vi "GatlingLoop.vi"(8 "error in":errorcluster) -> ()   [LabVIEW 2014]
uses:
  <vilib>/Rock Robotics/WPI/Relay/WPI_RelayValue.ctl
  <vilib>/Rock Robotics/WPI/Solenoid/WPI_SolenoidValue.ctl
  Robot Global Data.vi
  <vilib>/Rock Robotics/WPI/Solenoid/WPI_SolenoidSetEnum.vi
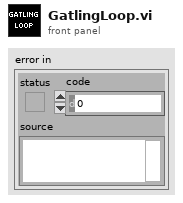
[diagram p1: front panel]
types:
  T1 = typedef "WPI_SolenoidValue.ctl" = enum16{"Off", "On", "Forward", "Reverse"}
  T2 = typedef "WPI_RelayValue.ctl" = enum16{"Off", "On", "Forward", "Reverse"}
  T3 = typedef "WPI_SolenoidDevRef.ctl" = cluster{"DevStatus":errorcluster, "Pneumatics Control Module":u8, "Forward Solenoid Channel":T4, "Reverse Solenoid Channel":T4}
  T4 = typedef "WPI_SolenoidChannel.ctl" = enum8{"Solenoid 0", "Solenoid 1", "Solenoid 2", "Solenoid 3", "Solenoid 4", "Solenoid 5", "Solenoid 6", "Solenoid 7", "Invalid"}
  T5 = typedef "WPI_MotorControlDeviceRef.ctl" = cluster{"DeviceStatus":errorcluster, "Type":T6, "PWM":cluster{"Controller":T7, "PWM Channel":T8, "DeadBand":T9}, "CAN":cluster{"Device Number":u8, "Control Mode":T10, "Semaphore":T11, "Max Vout":dbl, "TalonSRX Control Mode":T12}, "Invert":bool, "TransformRef":T13, "InvTransformRef":T13}
  T6 = typedef "WPI_MotorControlType.ctl" = enum16{"PWM", "CAN", "CANTalonSRX"}
  T7 = typedef "FPGA_TypedefDigitalModule.ctl" = enum16{"Controller 1"}
  T8 = typedef "FPGA_DIOPWMChannel.ctl" = enum8{"PWM 0", "PWM 1", "PWM 2", "PWM 3", "PWM 4", "PWM 5", "PWM 6", "PWM 7", "PWM 8", "PWM 9", "PWM MXP 0", "PWM MXP 1", "PWM MXP 2", "PWM MXP 3", "PWM MXP 4", "PWM MXP 5", "PWM MXP 6", "PWM MXP 7", "PWM MXP 8", "PWM MXP 9", "Invalid"}
  T9 = typedef "WPI_PWMDeadband.ctl" = cluster{"Name":string, "maxPositivePwm":i32, "minPositivePwm":i32, "centerPwm":i32, "maxNegativePwm":i32, "minNegativePwm":i32, "angularRange":u16}
  T10 = typedef "WPI_CANJaguar_ControlMode.ctl" = enum8{"Percent VBus", "Current", "Speed", "Position", "Voltage"}
  T11 = typedef "Semaphore RefNum" = refnum<k1>
  T12 = typedef "WPI_CANTalonSRX_APIControlMode.ctl" = enum8{"Percent VBus", "Speed", "Position", "Slave", "Unchanged / Invalid"}
  T13 = typedef "WPI_PWMTransform_ConPane.ctl" = refnum<vi>
  T14 = typedef "WPI_RelayDevRef.ctl" = cluster{"DevStatus":errorcluster, "Relay Channel":T15, "Controller":T7, "Relay Direction":T16}
  T15 = typedef "FPGA_DIORelayChannel.ctl" = enum8{"Relay 0", "Relay 1", "Relay 2", "Relay 3", "Invalid"}
  T16 = typedef "WPI_RelayDirection.ctl" = enum16{"Both directions", "Forward only", "Reverse only"}
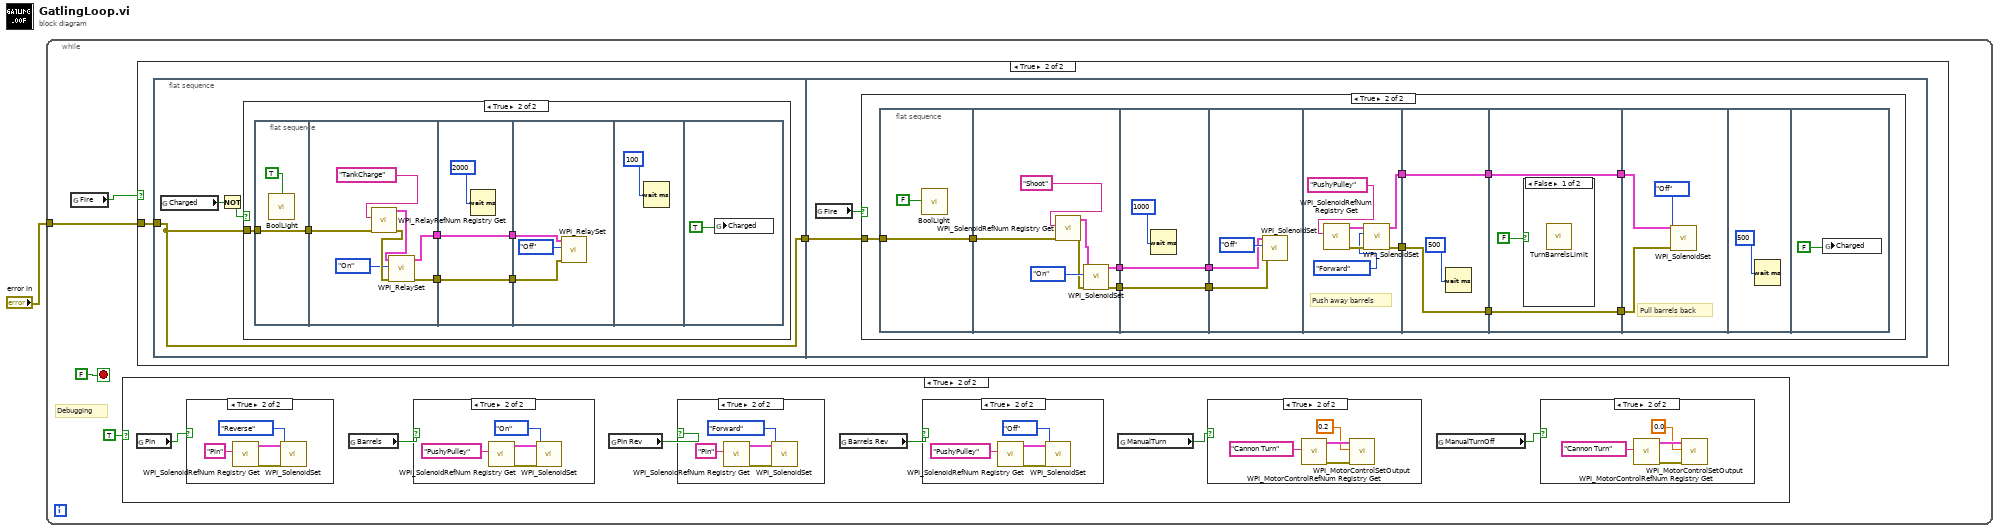
[diagram p0: block diagram]
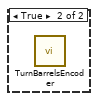
[diagram p12: hidden frame]
diagram:
  n1 = while {
    tunnel: "error in" -> [w3]
    stop <- FALSE stop-if-true
    # "Debugging"
    n2 = global read "Robot Global Data.vi" "Fire"() -> (w4:bool)
    n3 = case shown="True" TRUE {
      frame False {
      }
      frame True {
        n4 = global read "Robot Global Data.vi" "Pin"() -> (w11:bool)
        n5 = case shown="True" w11 {
          frame False {
          }
          frame True {
            n6 = call <vilib>:"WPI_SolenoidRefNum Registry Get.vi"("refnum name"="Pin") -> ("error out"=w34:errorcluster, "SolenoidDevRef"=w33:T3)  [unwired: 9 in]
            n7 = call-poly <vilib>:"WPI_SolenoidSet.vi"("error in (no error)"=w34, "Value"=WPI_SolenoidValue."Reverse", "SolenoidDevRef"=w33) -> ()  [unwired: 7 in, 2 out]
          }
        }
        n8 = global read "Robot Global Data.vi" "Barrels"() -> (w10:bool)
        n9 = case shown="True" w10 {
          frame False {
          }
          frame True {
            n10 = call <vilib>:"WPI_SolenoidRefNum Registry Get.vi"("refnum name"="PushyPulley") -> ("error out"=w30:errorcluster, "SolenoidDevRef"=w29:T3)  [unwired: 9 in]
            n11 = call-poly <vilib>:"WPI_SolenoidSet.vi"("error in (no error)"=w30, "Value"=WPI_SolenoidValue."On", "SolenoidDevRef"=w29) -> ()  [unwired: 7 in, 2 out]
          }
        }
        n12 = global read "Robot Global Data.vi" "Pin Rev"() -> (w9:bool)
        n13 = case shown="True" w9 {
          frame False {
          }
          frame True {
            n14 = call <vilib>:"WPI_SolenoidRefNum Registry Get.vi"("refnum name"="Pin") -> ("error out"=w26:errorcluster, "SolenoidDevRef"=w25:T3)  [unwired: 9 in]
            n15 = call-poly <vilib>:"WPI_SolenoidSet.vi"("error in (no error)"=w26, "Value"=WPI_SolenoidValue."Forward", "SolenoidDevRef"=w25) -> ()  [unwired: 7 in, 2 out]
          }
        }
        n16 = global read "Robot Global Data.vi" "Barrels Rev"() -> (w8:bool)
        n17 = case shown="True" w8 {
          frame False {
          }
          frame True {
            n18 = call <vilib>:"WPI_SolenoidRefNum Registry Get.vi"("refnum name"="PushyPulley") -> ("error out"=w22:errorcluster, "SolenoidDevRef"=w21:T3)  [unwired: 9 in]
            n19 = call-poly <vilib>:"WPI_SolenoidSet.vi"("error in (no error)"=w22, "Value"=WPI_SolenoidValue."Off", "SolenoidDevRef"=w21) -> ()  [unwired: 7 in, 2 out]
          }
        }
        n20 = global read "Robot Global Data.vi" "ManualTurn"() -> (w7:bool)
        n21 = case shown="True" w7 {
          frame False {
          }
          frame True {
            n22 = call <vilib>:"WPI_MotorControlRefNum Registry Get.vi"("refnum name"="Cannon Turn") -> ("error out"=w18:errorcluster, "MotorControlDevRef"=w17:T5)  [unwired: 9 in]
            n23 = call <vilib>:"WPI_MotorControlSetOutput.vi"("error in (no error)"=w18, "Output"=0.2, "MotorControlDevRef"=w17) -> ()  [unwired: 6 in, 3 out]
          }
        }
        n24 = global read "Robot Global Data.vi" "ManualTurnOff"() -> (w6:bool)
        n25 = case shown="True" w6 {
          frame False {
          }
          frame True {
            n26 = call <vilib>:"WPI_MotorControlRefNum Registry Get.vi"("refnum name"="Cannon Turn") -> ("error out"=w14:errorcluster, "MotorControlDevRef"=w13:T5)  [unwired: 9 in]
            n27 = call <vilib>:"WPI_MotorControlSetOutput.vi"("error in (no error)"=w14, "Output"=0.0, "MotorControlDevRef"=w13) -> ()  [unwired: 6 in, 3 out]
          }
        }
      }
    }
    n28 = case shown="True" w4 {
      tunnel: w3 -> [_ w37]
      frame False {
      }
      frame True {
        n29 = flat-sequence {
          tunnel: w37 -> [w38]
          tunnel: [w38] -> w36
          tunnel: w36 -> [w64]
          frame #0 {
            n30 = global read "Robot Global Data.vi" "Charged"() -> (w40:bool)
            n31 = Not(x=w40) -> (.not. x?=w39:bool)
            n32 = case shown="True" w39 {
              tunnel: w38 -> [_ w42]
              frame False {
              }
              frame True {
                n33 = flat-sequence {
                  tunnel: w42 -> [w48]
                  tunnel: [w48] -> w41
                  tunnel: [w51] -> w46
                  tunnel: [w50] -> w45
                  tunnel: w41 -> [w49]
                  tunnel: [w57] -> w44
                  tunnel: w46 -> [w57]
                  tunnel: [w56] -> w43
                  tunnel: w45 -> [w56]
                  tunnel: w44 -> [w60]
                  tunnel: w43 -> [w59]
                  frame #0 {
                    n34 = call "BoolLight.vi"("On"=TRUE) -> ()
                  }
                  frame #1 {
                    n35 = call <vilib>:"WPI_RelayRefNum Registry Get.vi"("error in (no error)"=w49, "refnum name"="TankCharge") -> ("error out"=w53:errorcluster, "RelayDevRef"=w54:T14)  [unwired: 8 in]
                    n36 = call <vilib>:"WPI_RelaySet.vi"("error in (no error)"=w53, "RelayValue"=WPI_RelayValue."On", "RelayDevRef"=w54) -> ("error out"=w50:errorcluster, "RelayDevRef"=w51:T14)  [unwired: 7 in]
                  }
                  frame #2 {
                    n37 = Wait (ms)(milliseconds to wait=u32 2000) -> ()  [unwired: 1 out]
                  }
                  frame #3 {
                    n38 = call <vilib>:"WPI_RelaySet.vi"("error in (no error)"=w59, "RelayValue"=WPI_RelayValue."Off", "RelayDevRef"=w60) -> ()  [unwired: 7 in, 2 out]
                  }
                  frame #4 {
                    n39 = Wait (ms)(milliseconds to wait=u32 100) -> ()  [unwired: 1 out]
                  }
                  frame #5 {
                    n40 = global write "Robot Global Data.vi" "Charged"(TRUE) -> ()
                  }
                }
              }
            }
          }
          frame #1 {
            n41 = global read "Robot Global Data.vi" "Fire"() -> (w65:bool)
            n42 = case shown="True" w65 {
              tunnel: w64 -> [_ w69]
              frame False {
              }
              frame True {
                n43 = flat-sequence {
                  tunnel: w69 -> [w79]
                  tunnel: [w79] -> w68
                  tunnel: [w82] -> w77
                  tunnel: [w81] -> w76
                  tunnel: w68 -> [w80]
                  tunnel: [w88] -> w75
                  tunnel: w77 -> [w88]
                  tunnel: [w87] -> w74
                  tunnel: w76 -> [w87]
                  tunnel: w75 -> [w91]
                  tunnel: w74 -> [w90]
                  tunnel: [w94] -> w73
                  tunnel: [w93] -> w72
                  tunnel: [w101] -> w67
                  tunnel: [w100] -> w66
                  tunnel: w72 -> [w100]
                  tunnel: w73 -> [w101]
                  tunnel: [w103] -> w71
                  tunnel: w67 -> [w103]
                  tunnel: [w102] -> w70
                  tunnel: w66 -> [w102]
                  tunnel: w71 -> [w107]
                  tunnel: w70 -> [w106]
                  frame #0 {
                    n44 = call "BoolLight.vi"("On"=FALSE) -> ()
                  }
                  frame #1 {
                    n45 = call <vilib>:"WPI_SolenoidRefNum Registry Get.vi"("error in (no error)"=w80, "refnum name"="Shoot") -> ("error out"=w83:errorcluster, "SolenoidDevRef"=w85:T3)  [unwired: 8 in]
                    n46 = call-poly <vilib>:"WPI_SolenoidSet.vi"("error in (no error)"=w83, "Value"=WPI_SolenoidValue."On", "SolenoidDevRef"=w85) -> ("error out"=w81:errorcluster, "SolenoidDevRef"=w82:T3)  [unwired: 7 in]
                  }
                  frame #2 {
                    n47 = Wait (ms)(milliseconds to wait=u32 1000) -> ()  [unwired: 1 out]
                  }
                  frame #3 {
                    n48 = call-poly <vilib>:"WPI_SolenoidSet.vi"("error in (no error)"=w90, "Value"=WPI_SolenoidValue."Off", "SolenoidDevRef"=w91) -> ()  [unwired: 7 in, 2 out]
                  }
                  frame #4 {
                    # "Push away barrels"
                    n49 = call <vilib>:"WPI_SolenoidRefNum Registry Get.vi"("refnum name"="PushyPulley") -> ("error out"=w97:errorcluster, "SolenoidDevRef"=w96:T3)  [unwired: 9 in]
                    n50 = call-poly <vilib>:"WPI_SolenoidSet.vi"("error in (no error)"=w97, "Value"=WPI_SolenoidValue."Forward", "SolenoidDevRef"=w96) -> ("error out"=w93:errorcluster, "SolenoidDevRef"=w94:T3)  [unwired: 7 in]
                  }
                  frame #5 {
                    n51 = Wait (ms)(milliseconds to wait=u32 500) -> ()  [unwired: 1 out]
                  }
                  frame #6 {
                    n52 = case shown="False" FALSE {
                      frame False {
                        n53 = call "TurnBarrelsLimit.vi"() -> ()  [unwired: 12 in]
                      }
                      frame True {
                        n54 = call "TurnBarrelsEncoder.vi"() -> ()  [unwired: 12 in]
                      }
                    }
                  }
                  frame #7 {
                    # "Pull barrels back"
                    n55 = call-poly <vilib>:"WPI_SolenoidSet.vi"("error in (no error)"=w106, "Value"=WPI_SolenoidValue."Off", "SolenoidDevRef"=w107) -> ()  [unwired: 7 in, 2 out]
                  }
                  frame #8 {
                    n56 = Wait (ms)(milliseconds to wait=u32 500) -> ()  [unwired: 1 out]
                  }
                  frame #9 {
                    n57 = global write "Robot Global Data.vi" "Charged"(FALSE) -> ()
                  }
                }
              }
            }
          }
        }
      }
    }
  }
